vi "getSubsystem.vi"(8 "error in (no error)":errorcluster, 10 "Name":string, 11 "Subsystem in":refnum<class "Subsystem.lvclass">) -> (0 "error out":errorcluster, 1 "Subsystem Found?":bool, 2 "Subsystem":refnum<class "Subsystem.lvclass">, 3 "Subsystem out":refnum<class "Subsystem.lvclass">)   [LabVIEW 2017, in "Subsystem.lvclass"]
uses:
  <userlib>/836-Library/Robot/Subsystem/Subsystem.lvclass
  <userlib>/836-Library/Robot/Subsystem/Subsystem.lvclass/Subsystem.ctl
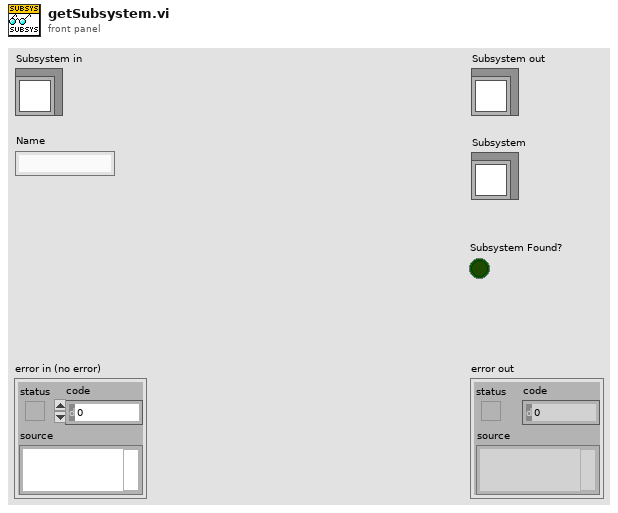
[diagram p1: front panel]
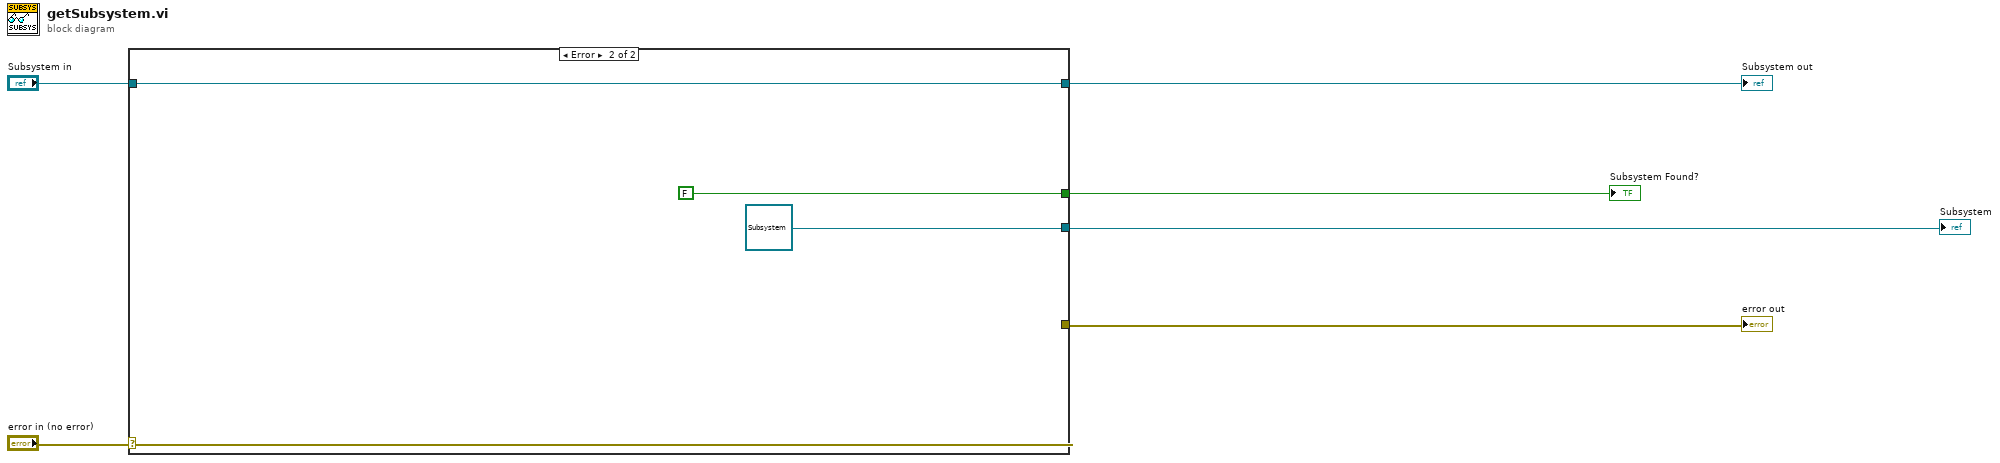
[diagram p0: block diagram]
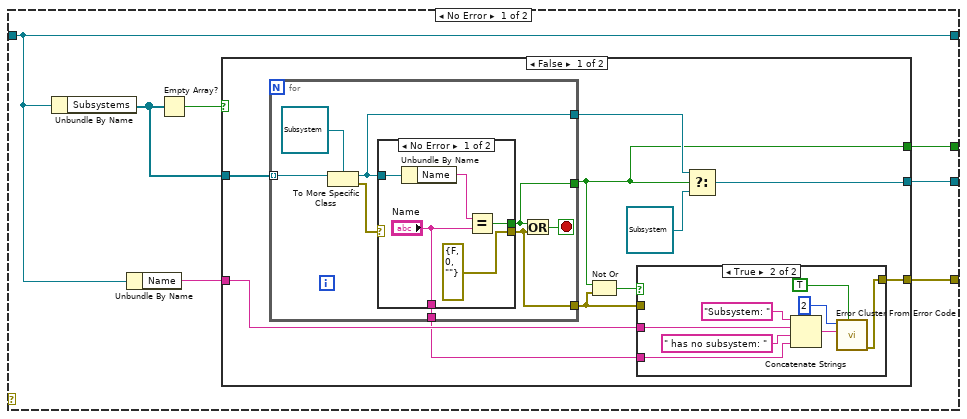
[diagram p2: hidden frame]
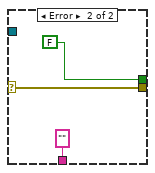
[diagram p4: hidden frame]
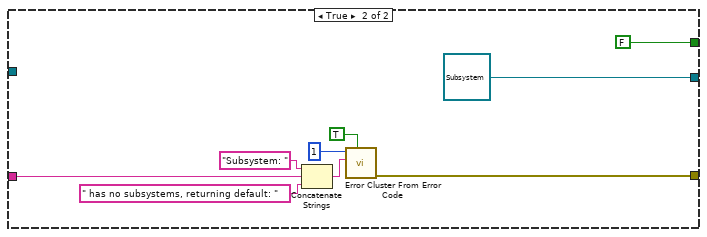
[diagram p5: hidden frame]
diagram:
  n1 = case shown="Error" "error in (no error)" {
    selector: "error in (no error)" -> [_ w60]
    tunnel: [w9 w60] -> w5
    tunnel: [w11 w61] -> w3
    tunnel: "Subsystem in" -> [w11 w61]
    tunnel: [w12 refnum<class "Subsystem.lvclass"> refnum ("Subsystem")] -> w2
    tunnel: [w7 FALSE] -> w1
    frame No Error {
      n2 = Unbundle By Name(w11) -> ("Subsystems"=w10:refnum<class>[])
      n3 = Unbundle By Name(w11) -> ("Name"=w8:string)
      n4 = Empty Array?(array=w10) -> (empty?=w13:bool)
      n5 = case shown="False" w13 {
        tunnel: [w20 refnum<class "Subsystem.lvclass"> refnum ("Subsystem")] -> w12
        tunnel: w10 -> [w23 _]
        tunnel: [w19 w51] -> w9
        tunnel: w8 -> [w15 w50]
        tunnel: [w17 FALSE] -> w7
        frame False {
          n6 = for {
            tunnel: w23 -> [w40] mode=indexing
            tunnel: [w36] -> w17
            tunnel: [w35] -> w22
            tunnel: [w34] -> w18
            tunnel: [w33] -> w14
            stop <- w37 stop-if-true
            n7 = To More Specific Class(target class=refnum<class "Subsystem.lvclass"> refnum ("Subsystem in"), reference=w40) -> (specific class reference=w35:refnum<class "Subsystem.lvclass">, error out=w38:errorcluster)  [unwired: 1 in]
            n8 = case shown="No Error" w38 {
              selector: w38 -> [_ w48]
              tunnel: w35 -> [w45 _]
              tunnel: [errorcluster {"status"=FALSE, "code"=0, "source"=""} ("error IO") w48] -> w34
              tunnel: [w43 FALSE] -> w36
              tunnel: ["Name" "" ("Name")] -> w33
              frame No Error {
                n9 = Unbundle By Name(w45) -> ("Name"=w44:string)
                n10 = Equal?(x=w44, y="Name") -> (x = y?=w43:bool)
              }
              frame Error {
              }
            }
            n11 = Or(x=w36, y=w34) -> (x .or. y?=w37:bool)
          }
          n12 = Not Or(1:w18, 2:w17) -> (0:w16:bool)
          n13 = case shown="True" w16 {
            tunnel: w18 -> [w24 _]
            tunnel: [w24 w32] -> w19
            tunnel: w15 -> [_ w28]
            tunnel: w14 -> [_ w26]
            frame False {
            }
            frame True {
              n14 = Concatenate Strings("Subsystem: ", w28, " has no subsystem: " ("string"), w26) -> (w25:string)
              n15 = call <vilib>:"Error Cluster From Error Code.vi"("show call chain? (False)"=TRUE, "error message (\"\")"=w25, "error code (0)"=2) -> ("error out"=w32:errorcluster)  [unwired: 6 in]
            }
          }
          n16 = Select(t=w22, s=w17, f=refnum<class "Subsystem.lvclass"> refnum) -> (s? t:f=w20:refnum<class "Subsystem.lvclass">)
        }
        frame True {
          n17 = Concatenate Strings("Subsystem: ", w50, " has no subsystems, returning default: ") -> (w54:string)
          n18 = call <vilib>:"Error Cluster From Error Code.vi"("show call chain? (False)"=TRUE, "error message (\"\")"=w54, "error code (0)"=1) -> ("error out"=w51:errorcluster)  [unwired: 6 in]
        }
      }
    }
    frame Error {
    }
  }
  "error out" <- w5
  "Subsystem out" <- w3
  "Subsystem" <- w2
  "Subsystem Found?" <- w1
